vi "Create Sine Wave LUT.vi"(7 "output level units":T1, 11 "sine wave properties":T2) -> (3 "Signal Properties":T3)   [LabVIEW 2021, in "DigitalAudioGenerationProcess.lvlib"]
uses:
  DigitalAudioGenerationProcess.lvlib
  <vilib>/PDM Acquisition Toolkit/host/Classes/Tasks/I2S Output/Control/SignalProperties.ctl
  <vilib>/PDM Acquisition Toolkit/host/Classes/Channels/I2S Ouput/Controls/GenerationChannelProperties.ctl
  controls/sine wave properties.ctl
  <vilib>/PDM Acquisition Toolkit/host/Classes/Channels/I2S Ouput/I2S Output Channel.lvclass
  <vilib>/PDM Acquisition Toolkit/host/Classes/Tasks/I2S Output/I2S Output Task.lvclass
  <vilib>/Analysis/NI_AALBase.lvlib
  controls/AudioGenTypeDefs.lvlib
  shared/controls/digital output level units.ctl
  shared/controls/audio controls.lvlib
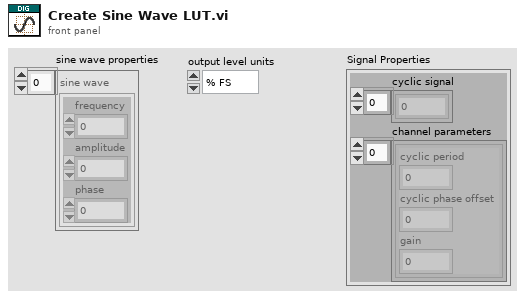
[diagram p1: front panel]
types:
  T1 = typedef "audio controls.lvlib/digital output level units.ctl" = enum32{"% FS", "dBFS", "V"}
  T2 = typedef "AudioGenTypeDefs.lvlib/sine wave properties.ctl" = cluster{"frequency":dbl, "amplitude":dbl, "phase":dbl}[]
  T3 = typedef "PDM Acquisition Class Library.lvlib/I2S Output Task.lvclass/SignalProperties.ctl" = cluster{"cyclic signal":dbl[], "channel parameters":T4[]}
  T4 = typedef "PDM Acquisition Class Library.lvlib/I2S Output Channel.lvclass/GenerationChannelProperties.ctl" = cluster{"cyclic period":dbl, "cyclic phase offset":dbl, "gain":dbl}
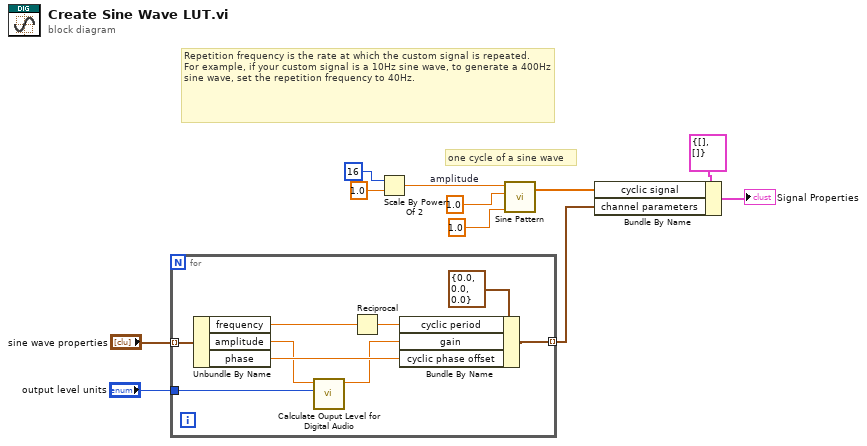
[diagram p0: block diagram]
diagram:
  w11 = 1.0  # amplitude
  # "one cycle of a sine wave"
  # "Repetition frequency is the rate at which the custom signal is repeated.\nFor example, if your custom signal is a 10Hz sine wave, to generate a 400Hz sine wave, set the repetition frequency to 40Hz."
  n1 = for {
    tunnel: "sine wave properties" -> [w18] mode=indexing
    tunnel: [w15] -> w2 mode=indexing
    tunnel: "output level units" -> [w12]
    n2 = Unbundle By Name(w18) -> ("frequency"=w17:dbl, "amplitude"=w14:dbl, "phase"=w16:dbl)
    n3 = call "Calculate Ouput Level for Digital Audio.vi"("digital output level units"=w12, "output level"=w14) -> ("gain"=w13:dbl)  [unwired: 8 in, 1 out]
    n4 = Reciprocal(x=w17) -> (1/x=w19:dbl)
    n5 = Bundle By Name(cluster=T4 {"cyclic period"=0.0, "cyclic phase offset"=0.0, "gain"=0.0}, "cyclic period"=w19, "gain"=w13, "cyclic phase offset"=w16) -> (w15:T4)
  }
  n6 = Scale By Power Of 2(n=i16 16, x=1.0) -> (x*2^n=w7:dbl)
  n7 = call <vilib>:"Sine Pattern.vi"("cycles"=1.0, "amplitude"=w11, "samples"=w7) -> ("Sinusoidal Pattern"=w8:dbl[])  [unwired: 1 in, 1 out]
  n8 = Bundle By Name(cluster=T3 {"cyclic signal"=[], "channel parameters"=[]} ("Signal Properties"), "cyclic signal"=w8, "channel parameters"=w2) -> (→"Signal Properties":T3)
